vi "XYZStage-Stop all movement command (ver 2).vi"(8 "Error In":errorcluster, 11 "XYZ Stage Control in":refnum<class "XYZ Stage Control.lvclass">) -> (0 "Error Out":errorcluster, 3 "XYZ Stage Control out":refnum<class "XYZ Stage Control.lvclass">)   [LabVIEW 2020]
uses:
  XYZ Stage Control/XYZ Stage Control.lvclass
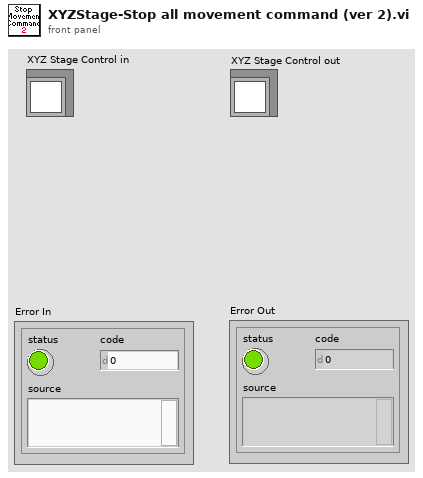
[diagram p1: front panel]
types:
  T1 = typedef "XYZ_position_input.ctl" = cluster{"Speed":i32, "Z Limit (um+/-)":sgl, "Axes":T2, "XYZ Coordinates":T3}
  T2 = typedef "XYZ axes.ctl" = string
  T3 = typedef "XYZ_coordinates.ctl" = cluster{"X":sgl, "Y":sgl, "Z":sgl}
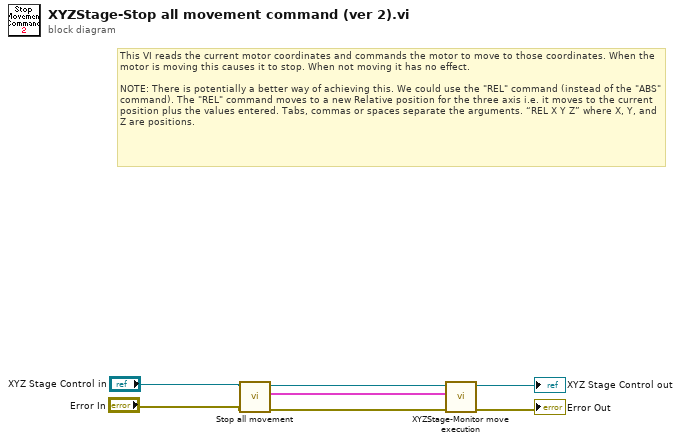
[diagram p0: block diagram]
diagram:
  # "This VI reads the current motor coordinates and commands the motor to move to those coordinates. When the motor is moving this causes it to stop. When not moving it has no effect.\n\nNOTE: There is potentially a better way of achieving this. We could use the \"REL\" command (instead of the \"ABS\" command). The \"REL\" command moves to a new Relative position for the three axis i.e. it moves to the current position plus the values entered. Tabs, commas or spaces separate the arguments. “REL X Y Z” where X, Y, and Z are positions."
  n1 = call-dynamic "Stop all movement.vi"("error in (no error)"="Error In", "XYZ Stage Control in"="XYZ Stage Control in") -> ("error out"=w5:errorcluster, "XYZ Position Set"=w4:T1, "XYZ Stage Control out"=w6:refnum<class "XYZ Stage Control.lvclass">)  [unwired: 7 in]
  n2 = call "XYZStage-Monitor move execution.vi"("error in (no error)"=w5, "XYZ Position Command Output"=w4, "XYZ Stage Control in"=w6) -> ("error out"=→"Error Out":errorcluster, "XYZ Stage Control out"=→"XYZ Stage Control out":refnum<class "XYZ Stage Control.lvclass">)  [unwired: 4 in, 3 out]
